vi "CAEN PSM Output DC Volts.vi"() -> ()   [LabVIEW 2017]
doc: "This example shows how to configure the instrument's output voltage level, over current protection, and over voltage protection. The actual voltage level and actual current level are returned as well as whether over voltage protection (OVP) or over current protection (OCP) has been tripped."
uses:
  <instrlib>/CAEN PSM/CAEN PSM.lvlib
panel:
  in  "Board family":u16(ring) items=["N/DT/NDT/R 14xx family", "DT55xxE familiy"]
  in  "Stop Output":bool
  out "OVC?":bool
  out "OVV?":bool
  in  "Voltage Max (0V)":dbl format="%.2f"
  out "Actual Current Limit (uA)":dbl format="%.2f"
  out "Actual Voltage Level (V)":dbl format="%.2f"
  in  "Voltage Level (0.0 V)":dbl format="%.2f"
  in  "Current Limit (0 uA)":dbl format="%.2f"
  in  "Channel":u8(ring) items=["Channel 0", "Channel 1", "Channel 2", "Channel 3"]
  in  "VISA resource name":refnum<visa-resource-name>
  # "(c) 2019 CAEN SpA.  ALL RIGHTS RESERVED."
  # "Adjust the settings before the run"
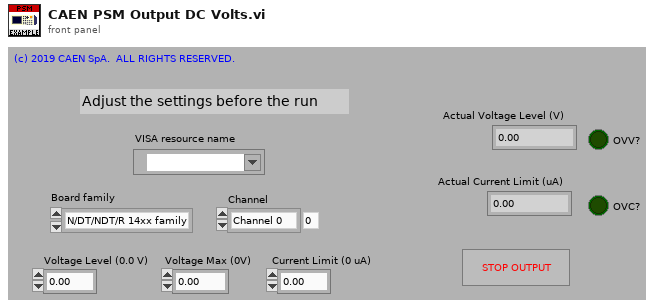
[diagram p1: front panel]
types:
  T1 = typedef "CAEN PSM.lvlib/BoardHandle.ctl" = cluster{"VISA resource name":refnum<visa-resource-name>, "Board address":i8, "NChannels":u8}
  T2 = cluster{"ON":bool, "RUP":bool, "RDW":bool, "OVC":bool, "OVV":bool, "UNV":bool, "MAXV":bool, "TRIP":bool, "OVP":bool, "OVT":bool, "DIS":bool, "KILL":bool, "ILK":bool, "NOCAL":bool}[]
  T3 = cluster{"ON":bool, "RUP":bool, "RDW":bool, "OVC":bool, "OVV":bool, "UNV":bool, "MAXV":bool, "TRIP":bool, "OVP":bool, "OVT":bool, "DIS":bool, "KILL":bool, "ILK":bool, "NOCAL":bool}
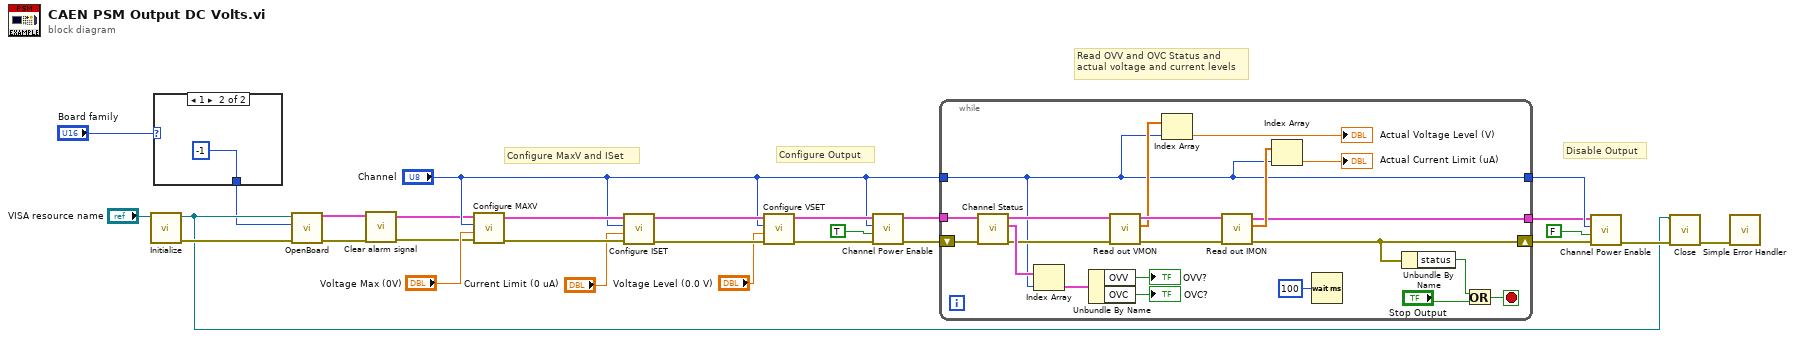
[diagram p0: block diagram]
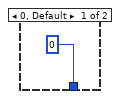
[diagram p2: hidden frame]
diagram:
  # "Disable Output"
  # "Read OVV and OVC Status and\nactual voltage and current levels"
  # "Configure Output"
  # "Configure MaxV and ISet"
  n1 = call <instrlib>:"Initialize.vi"("VISA resource name"="VISA resource name") -> ("error out"=w20:errorcluster, "VISA resource name out"=w8:refnum<visa-resource-name>)  [unwired: 9 in]
  n2 = case shown="1" "Board family" {
    tunnel: [i8 0 ("Board Address") i8 -1 ("Board Address")] -> w1
    frame 0, Default {
    }
    frame 1 {
    }
  }
  n3 = call <instrlib>:"OpenBoard.vi"("error in (no error)"=w20, "Board Address"=w1, "VISA resource name"=w8) -> ("error out"=w6:errorcluster, "BoardHandle"=w3:T1)  [unwired: 7 in]
  n4 = call <instrlib>:"Clear alarm signal.vi"("error in (no error)"=w6, "BoardHandle"=w3) -> ("error out"=w5:errorcluster, "BoardHandle out"=w4:T1)  [unwired: 8 in]
  n5 = call <instrlib>:"Configure MAXV.vi"("error in (no error)"=w5, "Voltage Max (0.0 V)"="Voltage Max (0V)", "Channel (0)"="Channel", "BoardHandle"=w4) -> ("error out"=w23:errorcluster, "BoardHandle out"=w19:T1)  [unwired: 6 in]
  n6 = call <instrlib>:"Configure ISET.vi"("error in (no error)"=w23, "Current Limit (0.00 uA)"="Current Limit (0 uA)", "Channel (0)"="Channel", "BoardHandle"=w19) -> ("error out"=w27:errorcluster, "BoardHandle out"=w17:T1)  [unwired: 6 in]
  n7 = call <instrlib>:"Configure VSET.vi"("error in (no error)"=w27, "Voltage Level (0.0 V)"="Voltage Level (0.0 V)", "Channel (0)"="Channel", "BoardHandle"=w17) -> ("error out"=w16:errorcluster, "BoardHandle out"=w13:T1)  [unwired: 6 in]
  n8 = call <instrlib>:"Channel Power Enable.vi"("error in (no error)"=w16, "Enable (OFF)"=TRUE, "Channel (0)"="Channel", "BoardHandle"=w13) -> ("error out"=w15:errorcluster, "BoardHandle out"=w14:T1)  [unwired: 6 in]
  n9 = while {
    tunnel: w14 -> [w51]
    tunnel: "Channel" -> [w32]
    tunnel: [w32] -> w21
    shift-right: [w38] -> w25
    shift-left: w15 -> [w50]
    tunnel: [w33] -> w7
    stop <- w49 stop-if-true
    n10 = call <instrlib>:"Channel Status.vi"("error in (no error)"=w50, "BoardHandle"=w51) -> ("error out"=w42:errorcluster, "Channel Status Array"=w46:T2, "BoardHandle out"=w41:T1)  [unwired: 6 in, 1 out]
    n11 = Index Array(array=w46, index=w32) -> (element=w45:T3)
    n12 = Unbundle By Name(w45) -> ("OVV"=→"OVV?":bool, "OVC"=→"OVC?":bool)
    n13 = call <instrlib>:"Read out VMON.vi"("error in (no error)"=w42, "BoardHandle"=w41) -> ("error out"=w39:errorcluster, "VMon values (V)"=w37:dbl[], "BoardHandle out"=w40:T1)  [unwired: 7 in]
    n14 = Index Array(array=w37, index=w32) -> (element=→"Actual Voltage Level (V)":dbl)
    n15 = call <instrlib>:"Read out IMON.vi"("error in (no error)"=w39, "BoardHandle"=w40) -> ("error out"=w38:errorcluster, "IMon values (uA)"=w34:dbl[], "BoardHandle out"=w33:T1)  [unwired: 6 in, 1 out]
    n16 = Index Array(array=w34, index=w32) -> (element=→"Actual Current Limit (uA)":dbl)
    n17 = Wait (ms)(milliseconds to wait=u32 100) -> ()  [unwired: 1 out]
    n18 = Unbundle By Name(w38) -> ("status"=w47:bool)
    n19 = Or(x=w47, y="Stop Output") -> (x .or. y?=w49:bool)
  }
  n20 = call <instrlib>:"Channel Power Enable.vi"("error in (no error)"=w25, "Enable (OFF)"=FALSE, "Channel (0)"=w21, "BoardHandle"=w7) -> ("error out"=w24:errorcluster)  [unwired: 6 in, 1 out]
  n21 = call <instrlib>:"Close.vi"("error in (no error)"=w24, "VISA resource name"=w8) -> ("error out"=w10:errorcluster)  [unwired: 9 in]
  n22 = call <vilib>:"Simple Error Handler.vi"("error in (no error)"=w10) -> ()  [unwired: 4 in, 5 out]
